vi "Settimeout.vi"(10 "Set_Val":T1) -> (3 "OneOfTemplate out":refnum<class "nixnet_grpc_ReadFrameRequest_timeout_enum.lvclass">)   [LabVIEW 2019, in "xnet-grpc_client.lvlib" / "nixnet_grpc_ReadFrameRequest_timeout_enum.lvclass"]
uses:
  nixnet_grpc_ReadFrameRequest_timeout_enum.lvclass
  nixnet_grpc_TimeOut.ctl
  nixnet_grpc_ReadFrameRequest_timeout_enum.lvclass/nixnet_grpc_ReadFrameRequest_timeout_enum.ctl
  xnet-grpc_client.lvlib
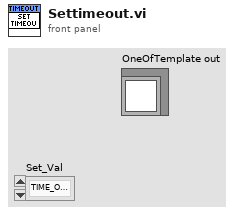
[diagram p1: front panel]
types:
  T1 = typedef "xnet-grpc_client.lvlib/nixnet_grpc_TimeOut.ctl" = enum32{"TIME_OUT_NONE", "TIME_OUT_INFINITE"}
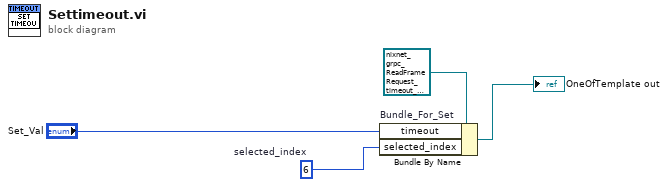
[diagram p0: block diagram]
diagram:
  w2 = 6  # selected_index
  n1 = Bundle By Name "Bundle_For_Set"(cluster=refnum<class "nixnet_grpc_ReadFrameRequest_timeout_enum.lvclass"> refnum ("OneOfTemplate in"), "timeout"="Set_Val", "selected_index"=w2) -> (→"OneOfTemplate out":refnum<class "nixnet_grpc_ReadFrameRequest_timeout_enum.lvclass">)
